vi "Data Reader.vi"   [LabVIEW 2024]
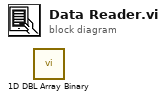
[diagram p0: block diagram]
diagram:
  n1 = call "1D DBL Array Binary.vi"() -> ()  [unwired: 11 in, 1 out]
